vi "Read Digital Data.vi"(8 "error in (no error)":errorcluster, 11 "Digital Write Single Msg in":refnum<class "Digital Write Single Msg.lvclass">) -> (0 "error out":errorcluster, 2 "Digital Data":bool, 3 "Digital Write Single Msg out":refnum<class "Digital Write Single Msg.lvclass">)   [LabVIEW 2024]
uses:
  Digital Write Single Msg.lvclass
  Digital Write Single Msg.lvclass/Digital Write Single Msg.ctl
  C:/Program Files (x86)/National Instruments/LabVIEW 2024/vi.lib/ActorFramework/Message/Message.lvclass
  C:/Users/uspoaotto/OneDrive - Oregon Tool/Desktop/working copies/DAQmxActor/src/DAQmx Actor/Digital Writer Messages/Digital Write Single Msg/Digital Write Single Msg.lvclass
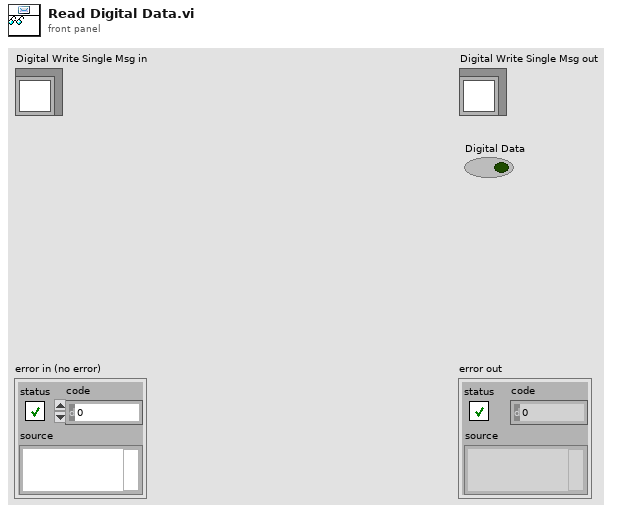
[diagram p1: front panel]
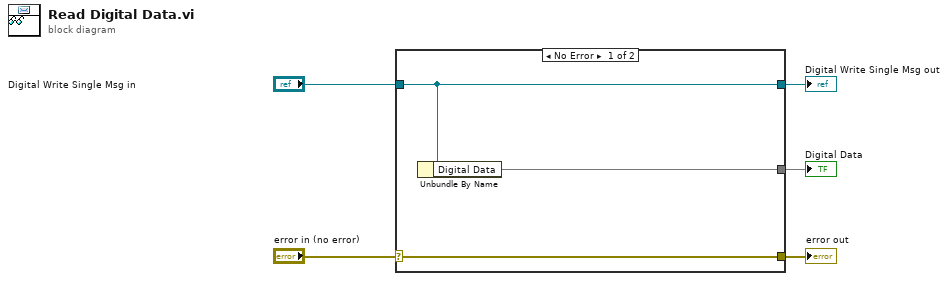
[diagram p0: block diagram]
diagram:
  n1 = case shown="No Error" "error in (no error)" {
    selector: "error in (no error)" -> [w8 w9]
    tunnel: [w8 w9] -> w4
    tunnel: [w7 w10] -> w2
    tunnel: "Digital Write Single Msg in" -> [w7 w10]
    tunnel: [w6 _] -> w1
    frame No Error {
      n2 = Unbundle By Name(w7) -> ("Digital Data"=w6)
    }
    frame Error {
    }
  }
  "error out" <- w4
  "Digital Write Single Msg out" <- w2
  "Digital Data" <- w1
